vi "Remove Software Feed.vi"(8 "error in (no error)":errorcluster, 10 "Feed Name":string, 11 "Session in":refnum<k21>) -> (0 "error out":errorcluster, 3 "Session out":refnum<k21>)   [LabVIEW 2020, in "nisyscfg.lvlib"]
doc: "Removes an existing software feed by name. This requires Secure Shell Server (sshd) to be enabled on the target."
uses:
  <vilib>/nisyscfg/nisyscfg.lvlib
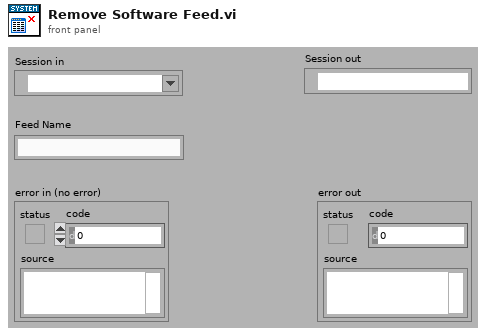
[diagram p1: front panel]
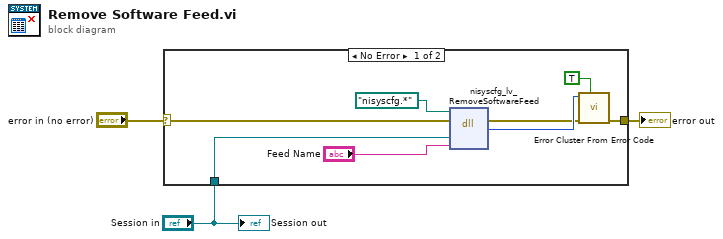
[diagram p0: block diagram]
diagram:
  n1 = case shown="No Error" "error in (no error)" {
    selector: "error in (no error)" -> [w6 w12]
    tunnel: [w7 w12] -> w3
    tunnel: "Session in" -> [w4 _]
    frame No Error {
      n2 = dll-call lib="nisyscfg.*" fn="nisyscfg_lv_RemoveSoftwareFeed" label="ModifySoftwareFeed"(path in=path "nisyscfg.*", error in=w6, "sessionHandle"=w4, "feedName"="Feed Name") -> (error out=w10:errorcluster, "return type"=w11:i32)  [unwired: 3 in, 1 out]
      n3 = call <vilib>:"Error Cluster From Error Code.vi"("show call chain? (False)"=TRUE, "error in (no error)"=w10, "error code (0)"=w11) -> ("error out"=w7:errorcluster)  [unwired: 6 out]
    }
    frame Error {
    }
  }
  "error out" <- w3
  "Session out" <- "Session in"
